vi "Arduino IR Sensor.vi"() -> ()   [LabVIEW 2011, in "LabVIEW Interface for Arduino.lvlib"]
doc: "An example that uses the Arduino with a IR sensor to detect movement. The example triggers an action when movement is seen and when movement stops being seen. The user can set a threshold for the number of seconds movement must be seen to trigger a movement action."
uses:
  <vilib>/LabVIEW Interface for Arduino/LabVIEW Interface for Arduino.lvlib
panel:
  in  "VISA resource name":refnum<visa-resource-name>
  in  "Stop":bool
  in  "Movement Limit (seconds)":dbl
  out "Movement Stopped Action":bool
  out "Movement Started Action":bool
  out "Movement Seen For(seconds)":dbl
  out "LastMovement":timestamp
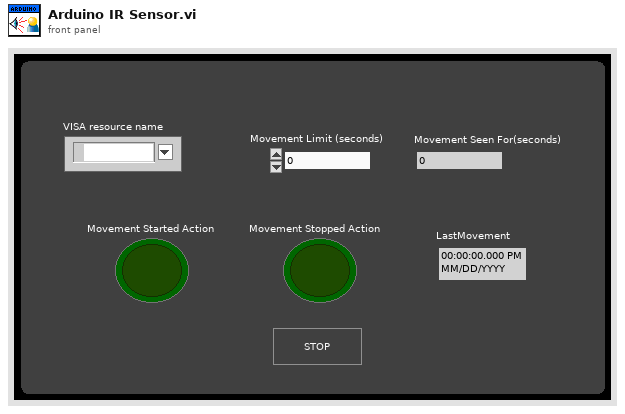
[diagram p1: front panel]
types:
  T1 = typedef "LabVIEW Interface for Arduino.lvlib/Arduino Resource.ctl" = cluster{"VISA resource":refnum<visa-resource-name>, "Board Type":T2, "Connection Type":enum8{"USB / Serial"}, "Bytes Per Packet (15)":u8}
  T2 = typedef "LabVIEW Interface for Arduino.lvlib/Board Type.ctl" = enum16{"Arduino Uno", "Dimuelanove w/Atmega 328", "Mega 2560", "Chipkit Uno32", "Chipkit Max32"}
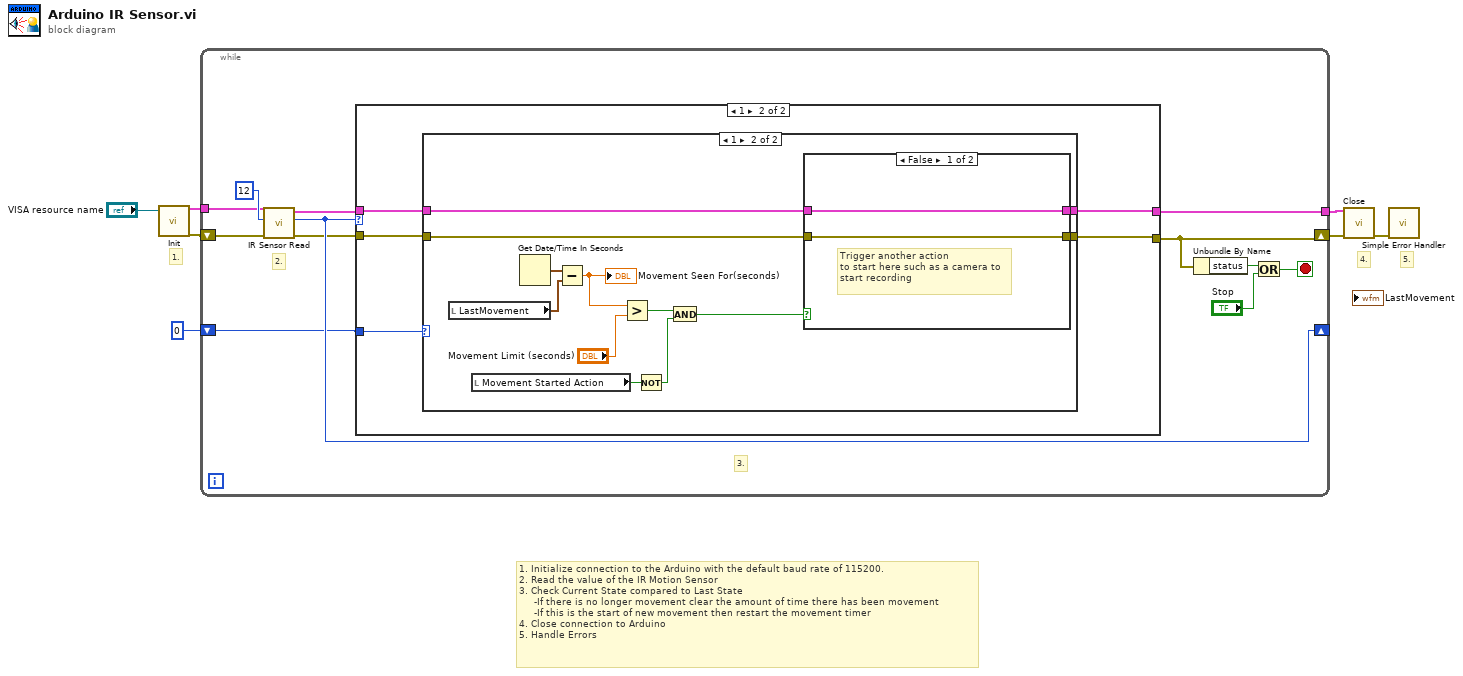
[diagram p0: block diagram]
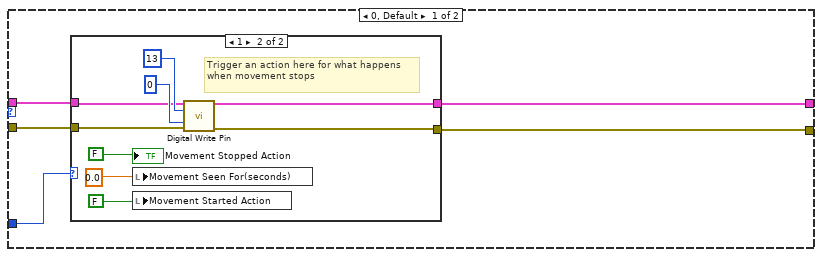
[diagram p2: hidden frame]
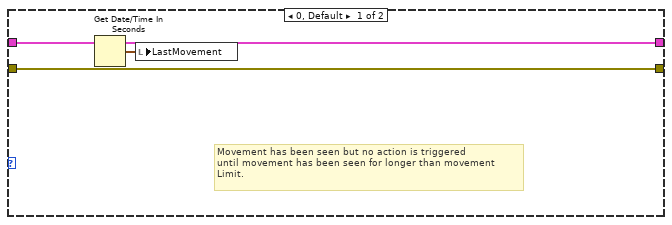
[diagram p4: hidden frame]
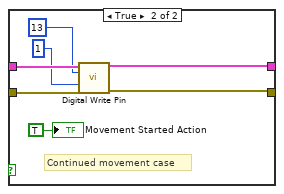
[diagram p5: hidden frame]
diagram:
  # "5."
  # "4."
  # "1."
  # "1. Initialize connection to the Arduino with the default baud rate of 115200.\n2. Read the value of the IR Motion Sensor\n3. Check Current State compared to Last State\n     -If there is no longer movement clear the amount of time there has been movement\n     -If this is the start of new movement then restart the movement timer\n4. Close connection to Arduino\n5. Handle Errors"
  n1 = call <vilib>:"Init.vi"("VISA resource"="VISA resource name") -> ("Arduino Resource"=w5:T1, "error out"=w7:errorcluster)  [unwired: 17 in]
  n2 = while {
    shift-right: [w8] -> w6
    shift-left: w7 -> [w18]
    tunnel: w5 -> [w13]
    shift-right: [w15] -> _
    shift-left: u8 0 ("MotionDetected") -> [w14]
    tunnel: [w11] -> w3
    stop <- w16 stop-if-true
    # "3."
    # "2."
    n3 = call <vilib>:"IR Sensor Read.vi"("error in"=w18, "Sensor Pin"=u8 12 ("Select DI Pin"), "Arduino Resource"=w13) -> ("error out"=w12:errorcluster, "MotionDetected"=w15:u8, "Arduino Resource"=w10:T1)  [unwired: 6 in]
    n4 = case shown="1" w15 {
      tunnel: w14 -> [w24 w40]
      tunnel: w12 -> [w23 w37]
      tunnel: [w22 w36] -> w8
      tunnel: [w21 w38] -> w11
      tunnel: w10 -> [w20 w39]
      frame 0, Default {
        n5 = case shown="1" w24 {
          tunnel: w23 -> [w25 w31]
          tunnel: [w25 w30] -> w22
          tunnel: [w26 w28] -> w21
          tunnel: w20 -> [w26 w27]
          frame 0, Default {
          }
          frame 1 {
            # "Trigger an action here for what happens\nwhen movement stops"
            n6 = local write "Movement Seen For(seconds)"(0.0 ("high for")) -> ()
            n7 = local write "Movement Started Action"(FALSE ("MovementStartedAction")) -> ()
            n8 = call <vilib>:"Digital Write Pin.vi"("Arduino Resource"=w27, "Digital I/O Pin (0)"=u8 13, "Value (0)"=u8 0, "error in"=w31) -> ("Arduino Resource"=w28:T1, "error out"=w30:errorcluster)  [unwired: 10 in]
            "Movement Stopped Action" <- FALSE ("MovementStoppedAction")
          }
        }
      }
      frame 1 {
        n9 = case shown="1" w40 {
          tunnel: w39 -> [w42 w47]
          tunnel: [w42 w46] -> w38
          tunnel: w37 -> [w41 w45]
          tunnel: [w41 w44] -> w36
          frame 0, Default {
            # "Movement has been seen but no action is triggered\nuntil movement has been seen for longer than movement\nLimit."
            n10 = Get Date/Time In Seconds() -> (seconds since 1Jan1904=w43:timestamp)
            n11 = local write "LastMovement"(w43) -> ()
          }
          frame 1 {
            n12 = local read "LastMovement"() -> (w54:timestamp)
            n13 = local read "Movement Started Action"() -> (w50:bool)
            n14 = Get Date/Time In Seconds() -> (seconds since 1Jan1904=w55:timestamp)
            n15 = Subtract(x=w55, y=w54) -> (x-y=w53:dbl)
            "Movement Seen For(seconds)" <- w53
            n16 = Greater?(x=w53, y="Movement Limit (seconds)") -> (0:w49:bool)
            n17 = Not(x=w50) -> (.not. x?=w51:bool)
            n18 = And(x=w49, y=w51) -> (x .and. y?=w48:bool)
            n19 = case shown="False" w48 {
              tunnel: w47 -> [w57 w63]
              tunnel: [w57 w62] -> w46
              tunnel: w45 -> [w56 w61]
              tunnel: [w56 w58] -> w44
              frame False {
                # "Trigger another action \nto start here such as a camera to\nstart recording"
              }
              frame True {
                # "Continued movement case"
                n20 = call <vilib>:"Digital Write Pin.vi"("Arduino Resource"=w63, "Digital I/O Pin (0)"=u8 13, "Value (0)"=u8 1, "error in"=w61) -> ("Arduino Resource"=w62:T1, "error out"=w58:errorcluster)  [unwired: 10 in]
                "Movement Started Action" <- TRUE ("MovementStartedAction")
              }
            }
          }
        }
      }
    }
    n21 = Unbundle By Name(w8) -> ("status"=w17:bool)
    n22 = Or(x=w17, y="Stop") -> (x .or. y?=w16:bool)
  }
  n23 = call <vilib>:"Close.vi"("Arduino Resource"=w3, "error in"=w6) -> ("error out"=w4:errorcluster)  [unwired: 13 in]
  n24 = call <vilib>:"Simple Error Handler.vi"("error in (no error)"=w4) -> ()  [unwired: 4 in, 5 out]
